vi "setDAQmx.AI_config.vi"(8 "error in (no error)":errorcluster, 10 "DAQmx.AI_Config":T1={"AI.Coupling"=10045, "input terminal configuration "=-1} {"input terminal configuration" items=["default"=-1, "RSE"=10083, "NRSE"=10078, "Differential"=10106, "Pseudodifferential"=12529]; "AI.Coupling" items=["AC"=10045, "DC"=10050, "GND"=10066]}, 11 "DAQmx.AI in":refnum<class "DAQmx.AI.lvclass">) -> (0 "error out":errorcluster, 3 "DAQmx.AI out":refnum<class "DAQmx.AI.lvclass">)   [LabVIEW 2020, in "DAQmx.AI.lvclass"]
uses:
  DAQmx.AI.lvclass
  Typedefs/DAQmx.AI_Config.ctl
  Typedefs/AI.Coupling-enum.ctl
  Typedefs/AI.Terminal-enum.ctl
  DAQmx.AI.lvclass/DAQmx.AI.ctl
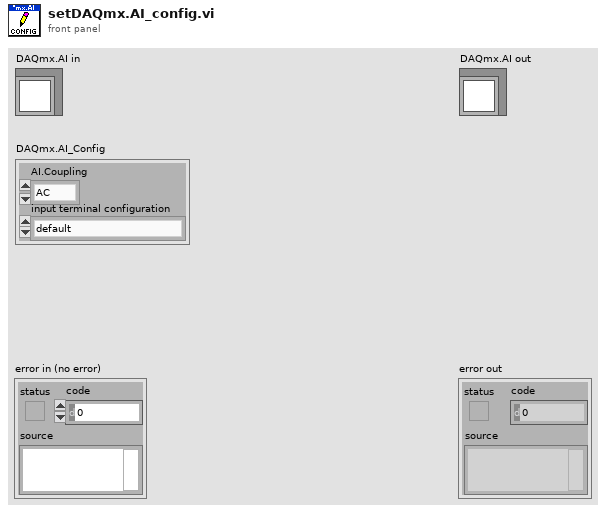
[diagram p1: front panel]
types:
  T1 = typedef "DAQmx.AI.lvclass/DAQmx.AI_Config.ctl" = cluster{"AI.Coupling":T2, "input terminal configuration ":T3}
  T2 = typedef "DAQmx.AI.lvclass/AI.Coupling-enum.ctl" = i32
  T3 = typedef "DAQmx.AI.lvclass/AI.Terminal-enum.ctl" = i32
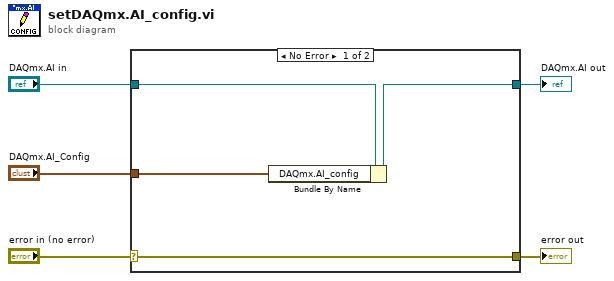
[diagram p0: block diagram]
diagram:
  n1 = case shown="No Error" "error in (no error)" {
    selector: "error in (no error)" -> [w9 w10]
    tunnel: [w9 w10] -> w4
    tunnel: [w7 w11] -> w2
    tunnel: "DAQmx.AI in" -> [w8 w11]
    tunnel: "DAQmx.AI_Config" -> [w6 _]
    frame No Error {
      n2 = Bundle By Name(cluster=w8, "DAQmx.AI_config"=w6) -> (w7:refnum<class "DAQmx.AI.lvclass">)
    }
    frame Error {
    }
  }
  "error out" <- w4
  "DAQmx.AI out" <- w2
